vi "Get DIO Channel Name.vi"(7 "DIO Channel Names":string[](array[string])=["A/DIO0", "A/DIO1", "A/DIO2", "A/DIO3", "A/DIO4", "A/DIO5", "A/DIO6", "A/DIO7", "A/DIO8", "A/DIO9", "A/DIO10", "A/DIO11", "A/DIO12", "A/DIO13", "A/DIO14", "A/DIO15", "B/DIO0", "B/DIO1", "B/DIO2", "B/DIO3", "B/DIO4", "B/DIO5", "B/DIO6", "B/DIO7", "B/DIO8", "B/DIO9", "B/DIO10", "B/DIO11", "B/DIO12", "B/DIO13", "B/DIO14", "B/DIO15", "C/DIO0", "C/DIO1", "C/DIO2", "C/DIO3", "C/DIO4", "C/DIO5", "C/DIO6", "C/DIO7"], 8 "Error In":errorcluster, 10 "DIO Channel Nums":u8[](array[numeric])) -> (0 "Error Out":errorcluster, 2 "DIO Channels":string[](array[string]))   [LabVIEW 2014, in "LMH-LINX.lvlib" / "myRIO.lvlib"]
doc: "Get DIO channel names (strings) from channel numbers."
uses:
  <vilib>/MakerHub/LINX/Private/myRIO/myRIO.lvlib
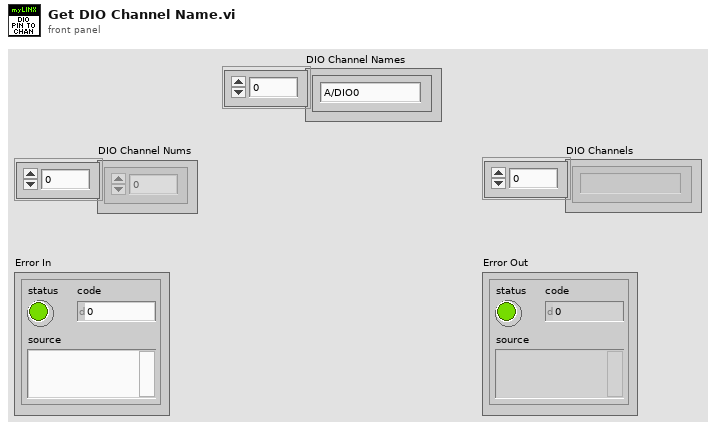
[diagram p1: front panel]
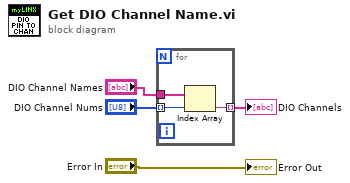
[diagram p0: block diagram]
diagram:
  n1 = for {
    tunnel: "DIO Channel Names" -> [w7]
    tunnel: "DIO Channel Nums" -> [w6] mode=indexing
    tunnel: [w5] -> w2 mode=indexing
    n2 = Index Array(array=w7, index=w6) -> (element=w5:string)
  }
  "DIO Channels" <- w2
  "Error Out" <- "Error In"
